vi "Truncate_cluster_Monitor.vi"(1 "Length":i32=20, 2 "System Monitor Variables":T1={"Time"=[], "LI1CH1"=[], "LI1CH2"=[], "LI2CH1"=[], "LI2CH2"=[], "LI3CH1"=[], "LI3CH2"=[], "Field"=[], "Temperature"=[], "Temperature 2"=[], "Temperatrue 3"=[], "Nitrogen_Level"=[], "Helium_Level"=[], "Heater_LS370"=[], "Sorb_Heater"=[], "Still_Heater"=[], "Capacity"=[], "Loss"=[], "Magnet_Temperature"=[], "Lambda_Pressure"=[], "Lambda_Needle_Valve"=[], "LS370-CH1-T"=[], "LS370-CH2-T"=[], "LS370-CH3-T"=[], "LS370-CH4-T"=[], "LS370-TC-T"=[], "LS370-CH1-R"=[], "LS370-CH2-R"=[], "LS370-CH3-R"=[], "LS370-CH4-R"=[], "LS370-TC-R"=[], "LS372-CH1-T"=[], "LS372-CH2-T"=[], "LS372-CH3-T"=[], "LS372-CH4-T"=[], "LS372-CH5-T"=[], "LS372-CH1-R"=[], "LS372-CH2-R"=[], "LS372-CH3-R"=[], "LS372-CH4-R"=[], "LS372-CH5-R"=[], "Nada"=[nan], "Keithley_Res"=[], "Keithley_Current"=[], "VTI_Heater"=[], "VTI_Needle Valve"=[], "LS340_Heater"=[], "Keithley_6221_Amplitude"=[], "Keithley_6221_Frequency"=[], "Condense_Pressure"=[], "Still_Pressure"=[], "FP_Out_Pressure"=[], "Dump_Pressure"=[], "V1"=[], "V2"=[], "V4"=[], "V5"=[], "V9"=[], "Forepump"=[], "Compressor"=[], "Keihtley_6221_Offset"=[], "BoxTemp"=[], "By"=[], "Bz"=[], "Phi"=[]}) -> (0 "System Monitor Variables 2":T1={"Time"=[], "LI1CH1"=[], "LI1CH2"=[], "LI2CH1"=[], "LI2CH2"=[], "LI3CH1"=[], "LI3CH2"=[], "Field"=[], "Temperature"=[], "Temperature 2"=[], "Temperatrue 3"=[], "Nitrogen_Level"=[], "Helium_Level"=[], "Heater_LS370"=[], "Sorb_Heater"=[], "Still_Heater"=[], "Capacity"=[], "Loss"=[], "Magnet_Temperature"=[], "Lambda_Pressure"=[], "Lambda_Needle_Valve"=[], "LS370-CH1-T"=[], "LS370-CH2-T"=[], "LS370-CH3-T"=[], "LS370-CH4-T"=[], "LS370-TC-T"=[], "LS370-CH1-R"=[], "LS370-CH2-R"=[], "LS370-CH3-R"=[], "LS370-CH4-R"=[], "LS370-TC-R"=[], "LS372-CH1-T"=[], "LS372-CH2-T"=[], "LS372-CH3-T"=[], "LS372-CH4-T"=[], "LS372-CH5-T"=[], "LS372-CH1-R"=[], "LS372-CH2-R"=[], "LS372-CH3-R"=[], "LS372-CH4-R"=[], "LS372-CH5-R"=[], "Nada"=[nan], "Keithley_Res"=[], "Keithley_Current"=[], "VTI_Heater"=[], "VTI_Needle Valve"=[], "LS340_Heater"=[], "Keithley_6221_Amplitude"=[], "Keithley_6221_Frequency"=[], "Condense_Pressure"=[], "Still_Pressure"=[], "FP_Out_Pressure"=[], "Dump_Pressure"=[], "V1"=[], "V2"=[], "V4"=[], "V5"=[], "V9"=[], "Forepump"=[], "Compressor"=[], "Keihtley_6221_Offset"=[], "BoxTemp"=[], "By"=[], "Bz"=[], "Phi"=[]})   [LabVIEW 2016]
uses:
  Global/Global Variables/System Monitor Cluster.ctl
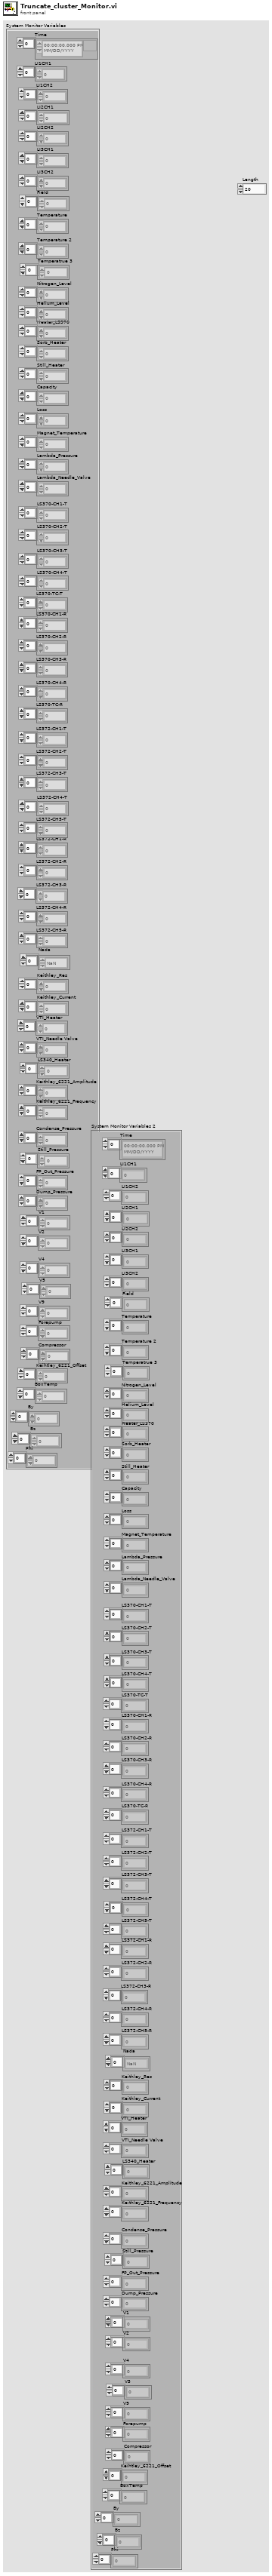
[diagram p1: front panel]
types:
  T1 = typedef "System Monitor Cluster.ctl" = cluster{"Time":timestamp[], "LI1CH1":dbl[], "LI1CH2":dbl[], "LI2CH1":dbl[], "LI2CH2":dbl[], "LI3CH1":dbl[], "LI3CH2":dbl[], "Field":dbl[], "Temperature":dbl[], "Temperature 2":dbl[], "Temperatrue 3":dbl[], "Nitrogen_Level":dbl[], "Helium_Level":dbl[], "Heater_LS370":dbl[], "Sorb_Heater":dbl[], "Still_Heater":dbl[], "Capacity":dbl[], "Loss":dbl[], "Magnet_Temperature":dbl[], "Lambda_Pressure":dbl[], "Lambda_Needle_Valve":dbl[], "LS370-CH1-T":dbl[], "LS370-CH2-T":dbl[], "LS370-CH3-T":dbl[], "LS370-CH4-T":dbl[], "LS370-TC-T":dbl[], "LS370-CH1-R":dbl[], "LS370-CH2-R":dbl[], "LS370-CH3-R":dbl[], "LS370-CH4-R":dbl[], "LS370-TC-R":dbl[], "LS372-CH1-T":dbl[], "LS372-CH2-T":dbl[], "LS372-CH3-T":dbl[], "LS372-CH4-T":dbl[], "LS372-CH5-T":dbl[], "LS372-CH1-R":dbl[], "LS372-CH2-R":dbl[], "LS372-CH3-R":dbl[], "LS372-CH4-R":dbl[], "LS372-CH5-R":dbl[], "Nada":dbl[], "Keithley_Res":dbl[], "Keithley_Current":dbl[], "VTI_Heater":dbl[], "VTI_Needle Valve":dbl[], "LS340_Heater":dbl[], "Keithley_6221_Amplitude":dbl[], "Keithley_6221_Frequency":dbl[], "Condense_Pressure":dbl[], "Still_Pressure":dbl[], "FP_Out_Pressure":dbl[], "Dump_Pressure":dbl[], "V1":dbl[], "V2":dbl[], "V4":dbl[], "V5":dbl[], "V9":dbl[], "Forepump":dbl[], "Compressor":dbl[], "Keihtley_6221_Offset":dbl[], "BoxTemp":dbl[], "By":dbl[], "Bz":dbl[], "Phi":dbl[]}
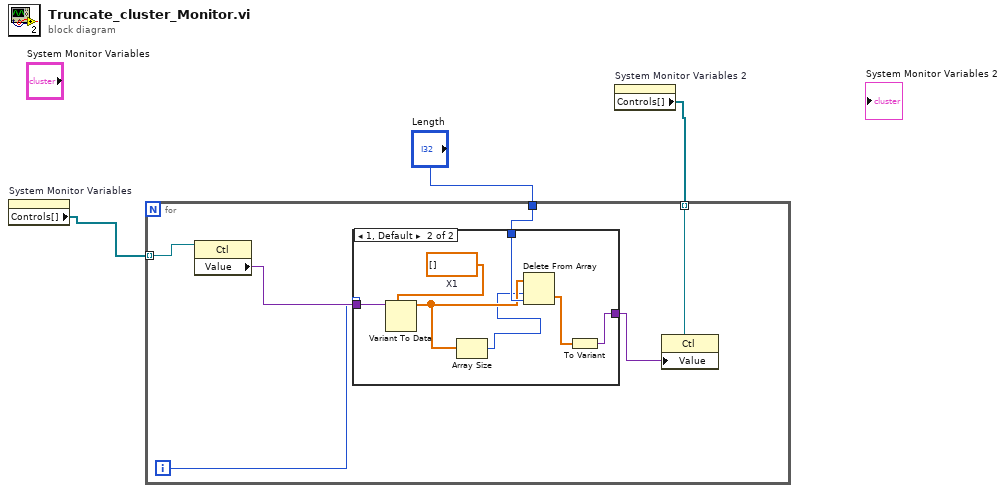
[diagram p0: block diagram]
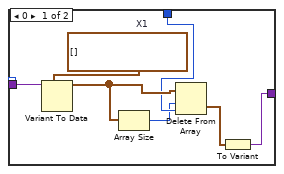
[diagram p2: hidden frame]
diagram:
  n1 = property on="System Monitor Variables" class="Clust (strict)"() -> ("Controls[]"=w2:refnum<vi>[])  [unwired: 2 in, 2 out]
  n2 = property on="System Monitor Variables 2" class="Clust (strict)"() -> ("Controls[]"=w1:refnum<vi>[])  [unwired: 2 in, 2 out]
  n3 = for {
    tunnel: w2 -> [w9] mode=indexing
    tunnel: "Length" -> [w5]
    tunnel: w1 -> [w7] mode=indexing
    i -> [w6]
    n4 = property class="Ctl"(reference=w9) -> ("Value"=w8:variant)  [unwired: 1 in, 2 out]
    n5 = case shown="1, Default" w6 {
      tunnel: w8 -> [w16 w23]
      tunnel: [w14 w21] -> w4
      tunnel: w5 -> [w12 w20]
      frame 0 {
        w15 = timestamp[] []  # X1
        n6 = Variant To Data(type=w15, Variant=w16) -> (data=w13:timestamp[])  [unwired: 1 in, 1 out]
        n7 = Array Size(array=w13) -> (size(s)=w10:i32)
        n8 = Delete From Array(array=w13, length=w10, index=w12) -> (deleted portion=w11:timestamp[])  [unwired: 1 out]
        n9 = To Variant(anything=w11) -> (Variant=w14:variant)
      }
      frame 1, Default {
        w22 = dbl[] []  # X1
        n10 = Variant To Data(type=w22, Variant=w23) -> (data=w19:dbl[])  [unwired: 1 in, 1 out]
        n11 = Array Size(array=w19) -> (size(s)=w17:i32)
        n12 = Delete From Array(array=w19, length=w17, index=w20) -> (deleted portion=w18:dbl[])  [unwired: 1 out]
        n13 = To Variant(anything=w18) -> (Variant=w21:variant)
      }
    }
    n14 = property class="Ctl"(reference=w7, "Value"=w4) -> ()  [unwired: 1 in, 2 out]
  }
